vi "sub_lidar_angle-inrange.vi"(7 "3d":bool, 8 "error in":errorcluster, 9 "2D data":cluster{"x":dbl, "y":dbl}[](array[cluster]), 10 "3D data":cluster{"x":dbl, "y":dbl, "z":dbl}[](array[cluster]), 11 "h range":cluster{"h-L":i16, "h-R":i16}) -> (0 "error out":errorcluster, 2 "xydata":cluster{"x":dbl, "y":dbl}[](array[cluster]), 3 "Array out":cluster{"x":dbl, "y":dbl}[](array[cluster]))   [LabVIEW 2019]
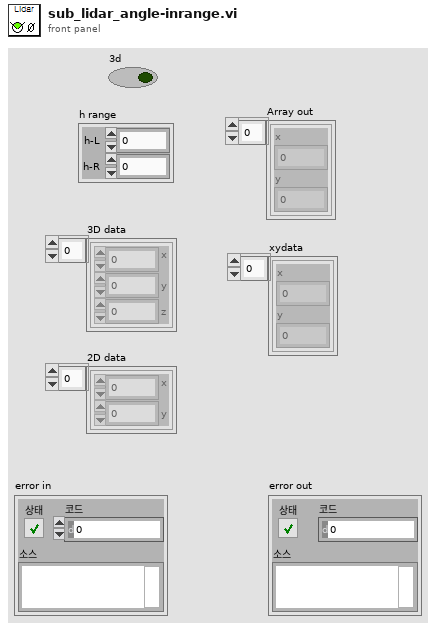
[diagram p1: front panel]
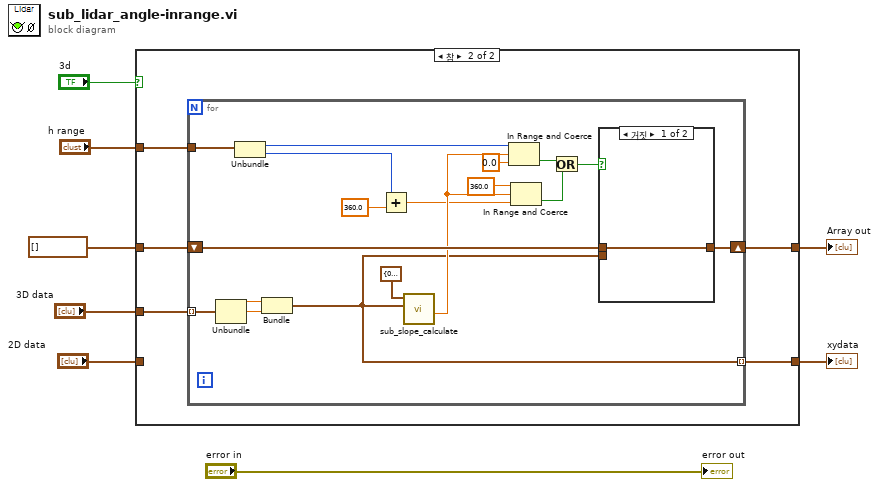
[diagram p0: block diagram]
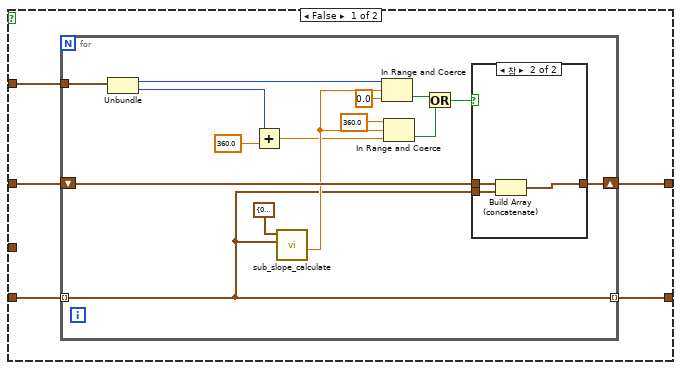
[diagram p2: hidden frame]
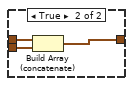
[diagram p4: hidden frame]
diagram:
  n1 = case shown="참" "3d" {
    tunnel: cluster{"x":dbl, "y":dbl}[] [] -> [w13 w36]
    tunnel: "h range" -> [w12 w37]
    tunnel: [w11 w34] -> w6
    tunnel: "3D data" -> [_ w35]
    tunnel: "2D data" -> [w10 _]
    tunnel: [w9 w33] -> w1
    frame False {
      n2 = for {
        shift-right: [w26] -> w11
        shift-left: w13 -> [w27]
        tunnel: w12 -> [w25]
        tunnel: w10 -> [w14] mode=indexing
        tunnel: [w14] -> w9 mode=indexing
        n3 = Unbundle(w25) -> ("h-L"=w24:i16, "h-R"=w20:i16)
        n4 = Add(x=w20, y=360.0) -> (x+y=w18:dbl)
        n5 = call "sub_slope_calculate.vi"("point n+1"=w14, "point n"=cluster{"x":dbl, "y":dbl} {"x"=0.0, "y"=0.0}) -> ("deg_gps-base"=w21:dbl)  [unwired: 7 in, 2 out]
        n6 = In Range and Coerce(upper limit=w24, x=w21, lower limit=0.0) -> (In Range?=w16:bool)  [unwired: 1 out]
        n7 = In Range and Coerce(upper limit=360.0 ("lower limit"), x=w21, lower limit=w18) -> (In Range?=w17:bool)  [unwired: 1 out]
        n8 = Or(x=w16, y=w17) -> (x .or. y?=w15:bool)
        n9 = case shown="참" w15 {
          tunnel: w27 -> [w29 w32]
          tunnel: [w29 w31] -> w26
          tunnel: w14 -> [_ w30]
          frame False {
          }
          frame True {
            n10 = Build Array (concatenate)(w32, w30) -> (w31:cluster{"x":dbl, "y":dbl}[])
          }
        }
      }
    }
    frame True {
      n11 = for {
        shift-right: [w51] -> w34
        shift-left: w36 -> [w52]
        tunnel: w37 -> [w50]
        tunnel: w35 -> [w39] mode=indexing
        tunnel: [w38] -> w33 mode=indexing
        n12 = Unbundle(w39) -> ("x"=w55:dbl, "y"=w54:dbl)  [unwired: 1 out]
        n13 = Unbundle(w50) -> ("h-L"=w49:i16, "h-R"=w45:i16)
        n14 = Bundle("x"=w55, "y"=w54) -> (w38:cluster{"x":dbl, "y":dbl})  [unwired: 1 in]
        n15 = Add(x=w45, y=360.0) -> (x+y=w43:dbl)
        n16 = call "sub_slope_calculate.vi"("point n+1"=w38, "point n"=cluster{"x":dbl, "y":dbl} {"x"=0.0, "y"=0.0}) -> ("deg_gps-base"=w46:dbl)  [unwired: 7 in, 2 out]
        n17 = In Range and Coerce(upper limit=w49, x=w46, lower limit=0.0) -> (In Range?=w41:bool)  [unwired: 1 out]
        n18 = In Range and Coerce(upper limit=360.0 ("lower limit"), x=w46, lower limit=w43) -> (In Range?=w42:bool)  [unwired: 1 out]
        n19 = Or(x=w41, y=w42) -> (x .or. y?=w40:bool)
        n20 = case shown="거짓" w40 {
          tunnel: w52 -> [w56 w59]
          tunnel: [w56 w58] -> w51
          tunnel: w38 -> [_ w57]
          frame False {
          }
          frame True {
            n21 = Build Array (concatenate)(w59, w57) -> (w58:cluster{"x":dbl, "y":dbl}[])
          }
        }
      }
    }
  }
  "Array out" <- w6
  "xydata" <- w1
  "error out" <- "error in"
